vi "Inst.Transport.TestLauncher.vi"() -> ()   [LabVIEW 2019, in "Inst.Transport.lvclass"]
uses:
  Inst.Transport.lvclass
  C:/Program Files/National Instruments/LabVIEW 2019/user.lib/LevyLab/Instrument Framework/Instrument/Instrument.lvclass
  C:/Program Files/National Instruments/LabVIEW 2019/vi.lib/JKI/JKI SMO/SMO/SMO.lvclass
  <vilib>/JKI/JKI SMO/SMO/SMO.lvclass/SMO.ctl
  <vilib>/JKI/JKI SMO/SMO/Typedefs/SMOState --Enum.ctl
  <vilib>/JKI/JKI SMO/SMO/Private/ReftoDVR--SMO.vi
  <userlib>/LevyLab/Instrument Framework/Instrument/Instrument.lvclass
  <vilib>/JKI/JKI SMO/SMO/SMO.lvclass
panel:
  in  "Hide":bool
  in  "Show":bool
  in  "Debug Mode? [F]":bool
  out "error out":errorcluster
  # "Example Instrument SMO Test Launcher"
  # "Close Panel to stop the SMO\n(press the \"X\")"
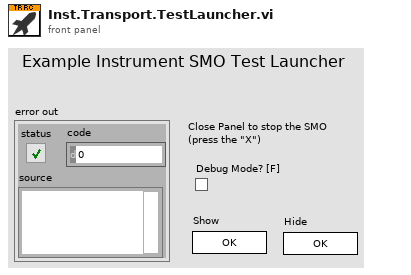
[diagram p1: front panel]
types:
  T1 = typedef "SMO.lvclass/Public Events.ctl" = cluster{"Error":refnum<user-event>, "State":refnum<user-event>, "Reserve State":refnum<user-event>}
  T2 = cluster{"Event Registration Refnum":refnum<event-registration>}
  T3 = typedef "SMO.lvclass/SMOState --Enum.ctl" = enum16{"unknown", "Created", "Started", "Stopped"}
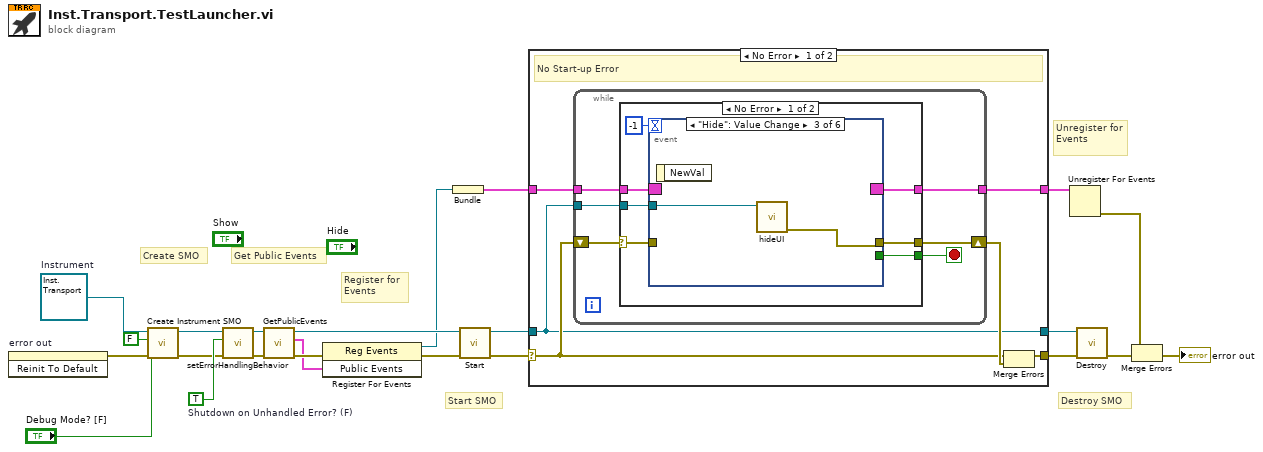
[diagram p0: block diagram]
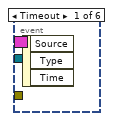
[diagram p2: hidden frame]
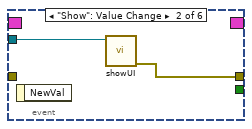
[diagram p3: hidden frame]
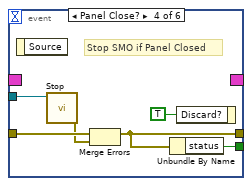
[diagram p4: hidden frame]
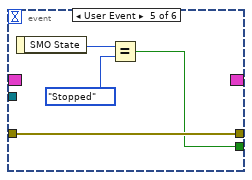
[diagram p5: hidden frame]
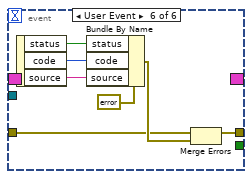
[diagram p6: hidden frame]
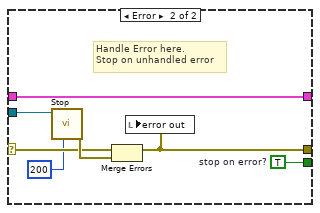
[diagram p7: hidden frame]
diagram:
  w5 = refnum<class "Inst.Transport.lvclass"> refnum  # Instrument
  w19 = TRUE  # Shutdown on Unhandled Error? (F)
  # "Get Public Events"
  # "Start SMO"
  # "Destroy SMO"
  # "Create SMO"
  # "Unregister for Events"
  # "Register for Events"
  n1 = invoke on="error out" class="Clust (strict)" method="Reinit To Default"() -> (error out=w6:errorcluster)  [unwired: 3 in, 2 out]
  n2 = call <userlib>:"Create Instrument SMO.vi"("error in (no error)"=w6, "Debug Mode? [F]"="Debug Mode? [F]", "Configuration Window? [T]"=FALSE, "Instrument in"=w5) -> ("error out"=w3:errorcluster, "Instrument out"=w4:refnum<class "Inst.Transport.lvclass">)  [unwired: 6 in]
  n3 = call <vilib>:"setErrorHandlingBehavior.vi"("error in (no error)"=w3, "Shutdown on Unhandled Error? (F)"=w19, "SMO in"=w4) -> ("error out"=w18:errorcluster, "SMO out"=w17:refnum<class "Inst.Transport.lvclass">)  [unwired: 7 in]
  n4 = call <vilib>:"GetPublicEvents.vi"("error in (no error)"=w18, "SMO"=w17) -> ("error out"=w15:errorcluster, "Public Events"=w14:T1, "SMO out"=w20:refnum<class "Inst.Transport.lvclass">)  [unwired: 7 in]
  n5 = register-events(error in=w15, w14) -> (reference out=w12:refnum<event-registration>, error out=w13:errorcluster)  [unwired: 1 in]
  n6 = Bundle("Event Registration Refnum"=w12) -> (w8:T2)  [unwired: 1 in]
  n7 = call <vilib>:"Start.vi"("error in (no error)"=w13, "SMO"=w20) -> ("error out"=w22:errorcluster, "SMO out"=w21:refnum<class "Inst.Transport.lvclass">)  [unwired: 8 in]
  n8 = case shown="No Error" w22 {
    selector: w22 -> [w25 w72]
    tunnel: [w29 w73] -> w7
    tunnel: w8 -> [w28 w73]
    tunnel: [w26 w72] -> w16
    tunnel: w21 -> [w24 w71]
    tunnel: [w24 w71] -> w23
    frame No Error {
      # "No Start-up Error"
      n9 = while {
        shift-right: [w34] -> w27
        shift-left: w25 -> [w30]
        tunnel: w28 -> [w33]
        tunnel: [w32] -> w29
        tunnel: w24 -> [w31]
        stop <- w35 stop-if-true
        n10 = case shown="No Error" w30 {
          selector: w30 -> [w37 w67]
          tunnel: [w42 w70] -> w35
          tunnel: [w41 w64] -> w34
          tunnel: w33 -> [w40 w69]
          tunnel: [w39 w69] -> w32
          tunnel: w31 -> [w38 w66]
          frame No Error {
            n11 = event shown="[2] \"Hide\": Value Change" {
              selector: w40 -> [_ _ _ _ _ _]
              dyn-events: [_ _ _ _ _ _] -> w39
              timeout: -1 -> [_ _ _ _ _ _]
              tunnel: [_ _ _ w50 w53 _] -> w42
              tunnel: w38 -> [_ w44 w46 w52 _ _]
              tunnel: [_ w43 w45 w47 w54 w57] -> w41
              tunnel: w37 -> [_ _ _ w49 w54 w58]
              event Timeout {
                n12 = event-data() -> ()  [unwired: 1 in, 3 out]
              }
              event "Show": Value Change {
                n13 = event-data() -> ()  [unwired: 1 in, 1 out]
                n14 = call "showUI.vi"("Inst.Transport in"=w44) -> ("error out"=w43:errorcluster)  [unwired: 9 in, 1 out]
              }
              event "Hide": Value Change {
                n15 = event-data() -> ()  [unwired: 1 in, 1 out]
                n16 = call "hideUI.vi"("Inst.Transport in"=w46) -> ("error out"=w45:errorcluster)  [unwired: 9 in, 1 out]
              }
              event Panel Close? {
                # "Stop SMO if Panel Closed"
                n17 = event-data() -> ()  [unwired: 1 in, 1 out]
                n18 = call <vilib>:"Stop.vi"("SMO"=w52) -> ("error out"=w48:errorcluster)  [unwired: 9 in, 1 out]
                n19 = Merge Errors(w49, w48) -> (w47:errorcluster)
                n20 = Unbundle By Name(w47) -> ("status"=w50:bool)
                n21 = event-data("Discard?"=TRUE ("OK")) -> ()  [unwired: 1 in, 1 out]
              }
              event User Event {
                n22 = event-data() -> ("SMO State"=w56:T3)  [unwired: 1 in]
                n23 = Equal?(x=w56, y=SMOState_--Enum."Stopped") -> (x = y?=w53:bool)
              }
              event User Event {
                n24 = event-data() -> ("status"=w63:bool, "code"=w62:i32, "source"=w61:string)  [unwired: 1 in]
                n25 = Bundle By Name(cluster=errorcluster {"status"=FALSE, "code"=0, "source"=""} ("error out"), "status"=w63, "code"=w62, "source"=w61) -> (w59:errorcluster)
                n26 = Merge Errors(w58, w59) -> (w57:errorcluster)
              }
            }
          }
          frame Error {
            w70 = TRUE  # stop on error?
            # "Handle Error here.\nStop on unhandled error"
            n27 = call <vilib>:"Stop.vi"("timeout in ms (-1)"=200, "SMO"=w66) -> ("error out"=w68:errorcluster)  [unwired: 8 in, 1 out]
            n28 = Merge Errors(w67, w68) -> (w64:errorcluster)
            n29 = local write "error out"(w64) -> ()
          }
        }
      }
      n30 = Merge Errors(w25, w27) -> (w26:errorcluster)
    }
    frame Error {
      # "Error occured before starting the process"
    }
  }
  n31 = Unregister For Events(event registration refnum=w7) -> (error out=w9:errorcluster)  [unwired: 1 in]
  n32 = call <vilib>:"Destroy.vi"("error in (no error)"=w16, "SMO"=w23) -> ("error out"=w11:errorcluster)  [unwired: 9 in]
  n33 = Merge Errors(w9, w11) -> (→"error out":errorcluster)
